vi "MatrixReset.vi"(8 "error in (no error)":errorcluster, 11 "GPIBSwitching in":refnum<class "GPIBSwitching.lvclass">) -> (0 "error out":errorcluster, 3 "GPIBSwitching out":refnum<class "GPIBSwitching.lvclass">)   [LabVIEW 2018, in "GPIBSwitching.lvclass"]
uses:
  GPIBSwitching.lvclass
  C:/ProbeTestSoftware2019/itk-strip-sensor-qc/InstrControl/InstrControl.lvclass
  Matrix_CommandsGlobal.vi
  InstrControl.lvclass
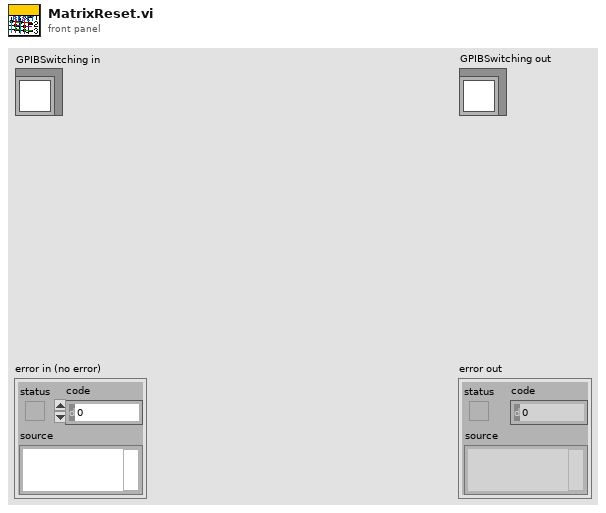
[diagram p1: front panel]
types:
  T1 = cluster{"Matrix address":string, "Instrument name":string, "Instrument type":u16, "Command \"Matrix Reset\"":string, "Command \"Connect Matrix Channels\"":string, "Command \"Disconnect Matrix Channels\"":string}
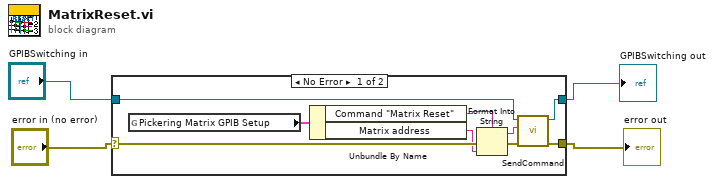
[diagram p0: block diagram]
diagram:
  n1 = case shown="No Error" "error in (no error)" {
    selector: "error in (no error)" -> [w10 w15]
    tunnel: [w5 w15] -> w2
    tunnel: [w12 w14] -> w1
    tunnel: "GPIBSwitching in" -> [w13 w14]
    frame No Error {
      n2 = global read "Matrix_CommandsGlobal.vi" "Pickering Matrix GPIB Setup"() -> (w11:T1)
      n3 = Unbundle By Name(w11) -> ("Command \"Matrix Reset\""=w8:string, "Matrix address"=w9:string)
      n4 = Format Into String(format string=w8, error in=w10, w9) -> (resulting string=w7:string, error out=w6:errorcluster)  [unwired: 1 in]
      n5 = call "SendCommand.vi"("error in (no error)"=w6, "Command string"=w7, "InstControl in"=w13) -> ("error out"=w5:errorcluster, "InstControl out"=w12:refnum<class "GPIBSwitching.lvclass">)  [unwired: 7 in]
    }
    frame Error {
    }
  }
  "error out" <- w2
  "GPIBSwitching out" <- w1
